vi "ATSpectrograph_Connect.vi"(8 "error in (no error)":errorcluster) -> (0 "error out":errorcluster, 3 "function return":i32)   [LabVIEW 2016, in "SALLV_ATSpectrograph.lvlib"]
doc: "int ATSpectrograph_salShmConnect();"
uses:
  SALLV_ATSpectrograph.lvlib
  SALLV_ATSpectrograph.so
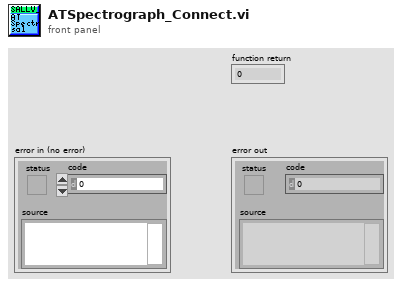
[diagram p1: front panel]
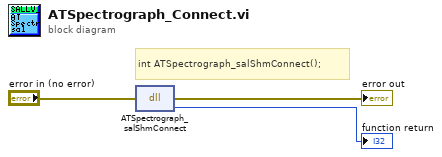
[diagram p0: block diagram]
diagram:
  # "int ATSpectrograph_salShmConnect();"
  n1 = dll-call lib="home/harini/tcs/SALLV_ATSpectrograph/SALLV_ATSpectrograph.*" fn="ATSpectrograph_salShmConnect"(error in="error in (no error)") -> (error out=→"error out":errorcluster, →"function return":i32)  [unwired: 2 in, 1 out]
